vi "matlab_script_run_2020.vi"() -> ()   [LabVIEW 2020]
panel:
  out "error out":errorcluster
  out "2-D Array of Real":dbl[][](array[numeric])
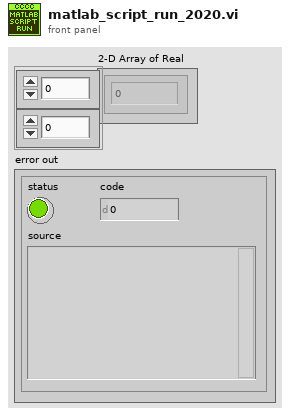
[diagram p1: front panel]
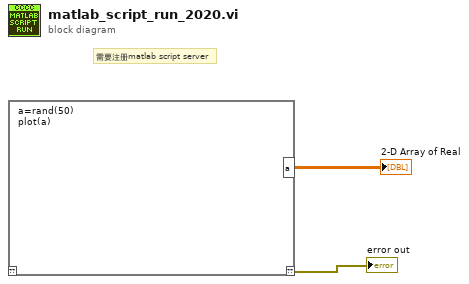
[diagram p0: block diagram]
diagram:
  # "需要注册matlab script server"
  n1 = script code="a=rand(50)\nplot(a)"() -> ("??"=→"error out":errorcluster, "a"=→"2-D Array of Real":dbl[][])  [unwired: 1 in]
